vi "Configure Multi Eval Meas Limit Power Dynamics Test Tolerances.vi"(7 "Power Great 3 GHz (0.0)":dbl format="%^.3e", 8 "error in (no error)":errorcluster, 9 "Power Less 3 GHz (0.0)":dbl format="%^.3e", 10 "Instance (1)":T1=1, 11 "VISA resource name":refnum<visa-resource-name>) -> (0 "error out":errorcluster, 3 "VISA resource name out":refnum<visa-resource-name>)   [LabVIEW 2020, in "Rohde&Schwarz CMWXP NR FR1 Measurement.lvlib"]
doc: "Defines test tolerances for power dynamics limits, for channel BW > 40 MHz.\n\nAttribute:\nRSCMWXPNRFR1M_ATTR_MULTI_EVAL_MEAS_LIMIT_POWER_DYNAMICS_TEST_TOLERANCES\n\nRemote-control command:\nCONFigure:NRSub:MEAS<i>:MEValuation:LIMit:PDYNamics:TTOLerance:CBGT"
uses:
  <instrlib>/Rohde&Schwarz CMWXP NR FR1 Measurement/Rohde&Schwarz CMWXP NR FR1 Measurement.lvlib
  <instrlib>/Rohde&Schwarz CMWXP NR FR1 Measurement/Private/_Instance.ctl
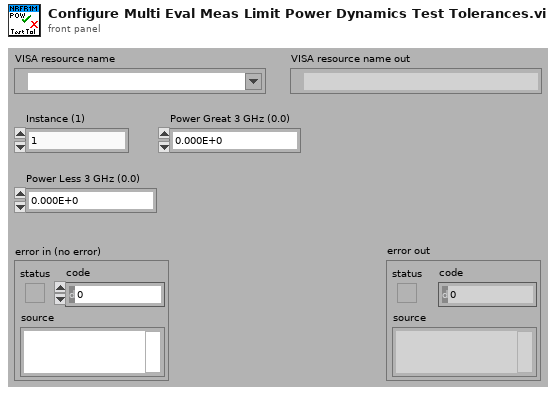
[diagram p1: front panel]
types:
  T1 = typedef "Rohde&Schwarz CMWXP NR FR1 Measurement.lvlib/_Instance.ctl" = i32
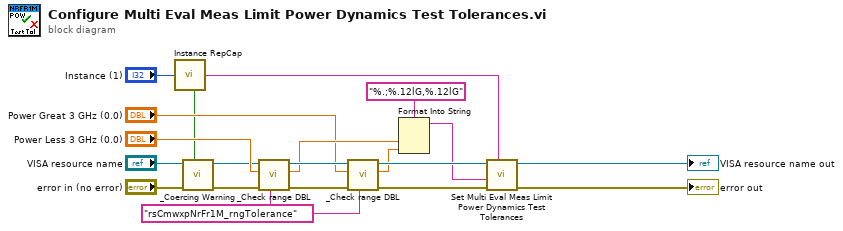
[diagram p0: block diagram]
diagram:
  w15 = "rsCmwxpNrFr1M_rngTolerance" ("Range Table Identifier")
  n1 = call <instrlib>:"Instance RepCap.vi"("Instance In"="Instance (1)") -> ("In Range?"=w1:bool, "RepCap Identifier Out"=w20:string)  [unwired: 1 in]
  n2 = call <instrlib>:"_Coercing Warning.vi"("In Range?"=w1, "error in (no error)"="error in (no error)", "VISA resource name"="VISA resource name") -> ("error out"=w3:errorcluster, "VISA resource name out"=w2:refnum<visa-resource-name>)  [unwired: 7 in]
  n3 = call <instrlib>:"_Check range DBL.vi"("Range Table Identifier"=w15, "error in (no error)"=w3, "DBL Value In"="Power Less 3 GHz (0.0)", "VISA resource name"=w2) -> ("error out"=w19:errorcluster, "DBL Value Out"=w13:dbl, "VISA resource name out"=w18:refnum<visa-resource-name>)  [unwired: 5 in]
  n4 = call <instrlib>:"_Check range DBL.vi"("Range Table Identifier"=w15, "error in (no error)"=w19, "DBL Value In"="Power Great 3 GHz (0.0)", "VISA resource name"=w18) -> ("error out"=w17:errorcluster, "DBL Value Out"=w12:dbl, "VISA resource name out"=w16:refnum<visa-resource-name>)  [unwired: 5 in]
  n5 = Format Into String(format string="%.;%.12lG,%.12lG", w13, w12) -> (resulting string=w11:string)  [unwired: 2 in, 1 out]
  n6 = call "Set Multi Eval Meas Limit Power Dynamics Test Tolerances"("Repeated Capabilities"=w20, "error in (no error)"=w17, "Multi Eval Meas Limit Power Dynamics Test Tolerances ()"=w11, "instrument handle"=w16) -> ("error out"=→"error out":errorcluster, "instrument handle out"=→"VISA resource name out":refnum<visa-resource-name>)  [unwired: 6 in]
